vi "Timer.vi"(11 "Previous_ms":u32) -> (1 "freq (hz)":dbl, 2 "dt (ms)":u32, 3 "Next_ms":u32)   [LabVIEW 2018]
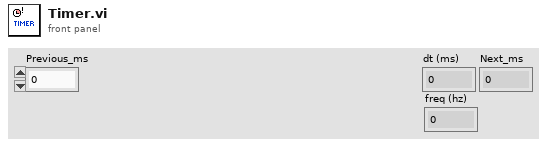
[diagram p1: front panel]
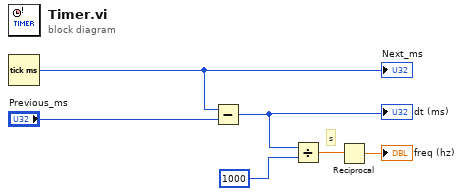
[diagram p0: block diagram]
diagram:
  # "s"
  n1 = Tick Count (ms)() -> (millisecond timer value=w6:u32)
  "Next_ms" <- w6
  n2 = Subtract(x=w6, y="Previous_ms") -> (x-y=w3:u32)
  "dt (ms)" <- w3
  n3 = Divide(x=w3, y=u32 1000) -> (x/y=w1:dbl)
  n4 = Reciprocal(x=w1) -> (1/x=→"freq (hz)":dbl)
